vi "EstimateGamePiece2.vi"(7 "piece?":enum16{"None", "Cube", "Cone"}(ring), 9 "Confidence":dbl, 11 "Vision Timestamp (ms)":u32, 12 "Gamepiece Y":dbl, 13 "Gamepiece X":dbl, 14 "Vision Valid?":bool, 15 "Range":dbl) -> (8 "Seen_Game_Pieces":T1(array[cluster]))   [LabVIEW 2020]
uses:
  GlobalPoseAndTargeting.vi
  GlobalArm.vi
panel:
  in  "Acceptable Radius":dbl=5.0 format="%#_13g"
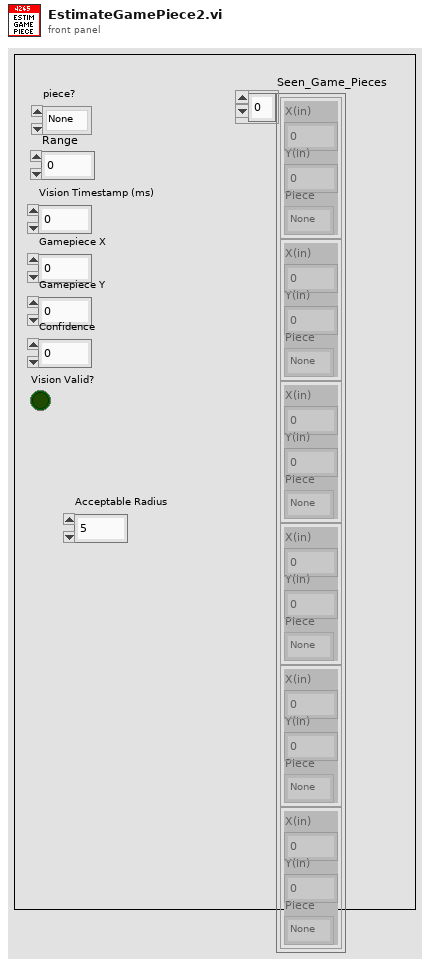
[diagram p1: front panel]
types:
  T1 = cluster{"X(in)":dbl, "Y(in)":dbl, "Piece":enum16{"None", "Cube", "Cone"}}[]
  T2 = cluster{"X":dbl, "Y":dbl, "Vision Timestamp (ms)":u32, "Confidence":dbl, "Range":dbl, "Piece":enum16{"None", "Cube", "Cone"}}
  T3 = cluster{"X":dbl, "Y":dbl, "Vision Timestamp (ms)":u32, "Confidence":dbl, "Range":dbl, "Piece":enum16{"None", "Cube", "Cone"}}[]
  T4 = cluster{"X(in)":dbl, "Y(in)":dbl, "Count":i32, "Timestamp(ms)":u32, "Piece":enum16{"None", "Cube", "Cone"}}
  T5 = cluster{"X(in)":dbl, "Y(in)":dbl, "Piece":enum16{"None", "Cube", "Cone"}}
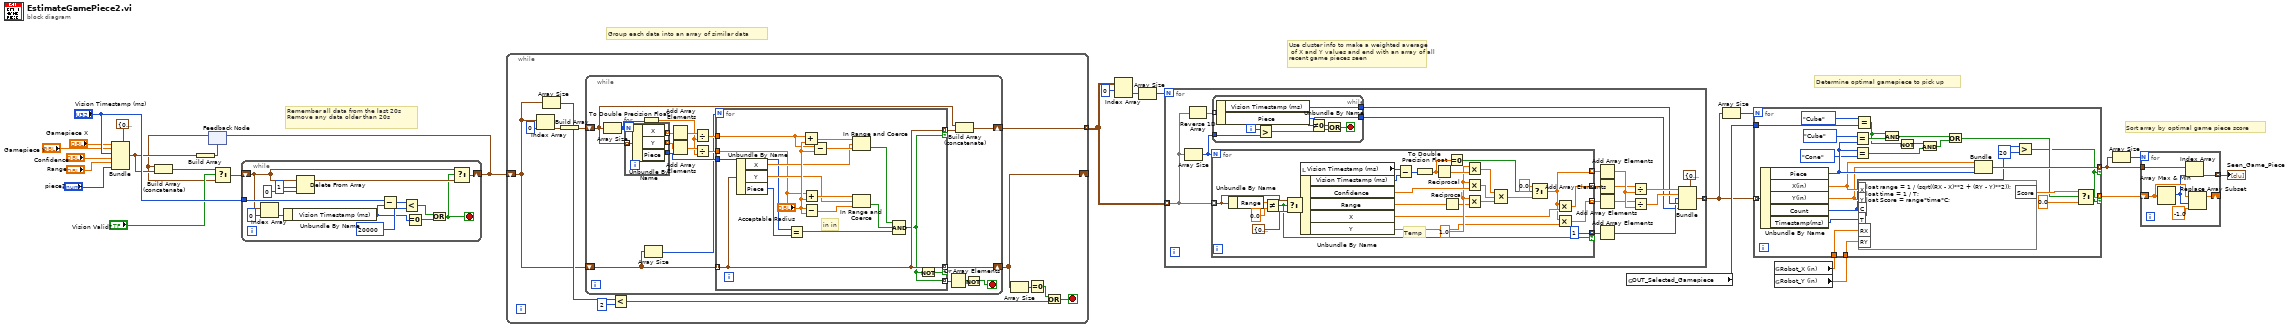
[diagram p0: block diagram]
diagram:
  # "Sort array by optimal game piece score"
  # "Determine optimal gamepiece to pick up"
  # "Use cluster info to make a weighted average\n of X and Y values and end with an array of all recent game pieces seen"
  # "Group each data into an array of similar data"
  # "Remember all data from the last 20s\nRemove any data older than 20s"
  n1 = Bundle(cluster=T2 {"X"=0.0, "Y"=0.0, "Vision Timestamp (ms)"=0, "Confidence"=0.0, "Range"=1.0, "Piece"=enum."None"} ("Cluster"), "X"="Gamepiece X", "Y"="Gamepiece Y", "Vision Timestamp (ms)"="Vision Timestamp (ms)", "Confidence"="Confidence", "Range"="Range", "Piece"="piece?") -> (w14:T2)
  n2 = Build Array(w14) -> (w13:T3)
  n3 = feedback #1(w13) -> (w2:T3)
  n4 = Build Array (concatenate)(w2, w14) -> (w4:T3)
  n5 = Select(t=w4, s="Vision Valid?", f=w2) -> (s? t:f=w5:T3)
  n6 = while {
    tunnel: "Vision Timestamp (ms)" -> [w39]
    shift-right: [w32] -> w1
    shift-left: w5 -> [w34]
    stop <- w28 stop-if-true
    n7 = Index Array(array=w34, index=0) -> (element=w40:T2)
    n8 = Unbundle By Name(w40) -> ("Vision Timestamp (ms)"=w31:u32)
    n9 = Delete From Array(array=w34, length=1, index=0) -> (array with subset deleted=w33:T3)  [unwired: 1 out]
    n10 = Subtract(x=w39, y=w31) -> (x-y=w38:u32)
    n11 = Less?(x=w38, y=u32 20000) -> (x < y?=w29:bool)
    n12 = Equal To 0?(x=w31) -> (x = 0?=w30:bool)
    n13 = Or(x=w29, y=w30) -> (x .or. y?=w28:bool)
    n14 = Select(t=w34, s=w28, f=w33) -> (s? t:f=w32:T3)
  }
  n15 = feedback-in #1(w1) -> ()
  n16 = while {
    shift-right: [w42] -> _
    shift-left: w1 -> [w46]
    tunnel: [w43] -> w11 mode=indexing
    stop <- w49 stop-if-true
    n17 = Index Array(array=w46, index=0) -> (element=w45:T2)
    n18 = Array Size(array=w46) -> (size(s)=w52:i32)
    n19 = Build Array(w45) -> (w44:T3)
    n20 = while {
      shift-right: [w62] -> w42
      shift-left: w46 -> [w55]
      shift-right: [w59] -> w43
      shift-left: w44 -> [w60]
      stop <- w56 stop-if-true
      n21 = Array Size(array=w60) -> (size(s)=w66:i32)
      n22 = for {
        N: w66 -> [_]
        tunnel: w60 -> [w75] mode=indexing
        tunnel: [w74] -> w71 mode=indexing
        tunnel: [w73] -> w70 mode=indexing
        tunnel: [w72] -> w69
        n23 = Unbundle By Name(w75) -> ("X"=w74:dbl, "Y"=w73:dbl, "Piece"=w72:enum16{"None", "Cube", "Cone"})
      }
      n24 = To Double Precision Float(number=w66) -> (double precision float=w63:dbl)
      n25 = Array Size(array=w55) -> (size(s)=w54:i32)
      n26 = Add Array Elements(numeric array=w71) -> (sum=w67:dbl)
      n27 = Add Array Elements(numeric array=w70) -> (sum=w65:dbl)
      n28 = Divide(x=w67, y=w63) -> (x/y=w68:dbl)
      n29 = Divide(x=w65, y=w63) -> (x/y=w64:dbl)
      n30 = for {
        N: w54 -> [_]
        tunnel: w55 -> [w80] mode=indexing
        tunnel: [w80] -> w61 mode=indexing if=w76
        tunnel: [w80] -> w62 mode=indexing if=w81
        tunnel: w68 -> [w79]
        tunnel: w64 -> [w78]
        tunnel: w69 -> [w77]
        tunnel: [w76] -> w58 mode=indexing
        # "in in"
        n31 = Unbundle By Name(w80) -> ("X"=w82:dbl, "Y"=w83:dbl, "Piece"=w84:enum16{"None", "Cube", "Cone"})
        n32 = Equal?(x=w77, y=w84) -> (x = y?=w85:bool)
        n33 = Add(x=w79, y="Acceptable Radius") -> (x+y=w92:dbl)
        n34 = Add(x=w78, y="Acceptable Radius") -> (x+y=w90:dbl)
        n35 = Subtract(x=w78, y="Acceptable Radius") -> (x-y=w89:dbl)
        n36 = Subtract(x=w79, y="Acceptable Radius") -> (x-y=w91:dbl)
        n37 = In Range and Coerce(upper limit=w92, x=w82, lower limit=w91) -> (In Range?=w87:bool)  [unwired: 1 out]
        n38 = In Range and Coerce(upper limit=w90, x=w83, lower limit=w89) -> (In Range?=w86:bool)  [unwired: 1 out]
        n39 = Compound Arithmetic op=AND(w87, w86, w85) -> (w76:bool)
        n40 = Not(x=w76) -> (.not. x?=w81:bool)
      }
      n41 = Or Array Elements(Boolean array=w58) -> (logical OR=w57:bool)
      n42 = Build Array (concatenate)(w60, w61) -> (w59:T3)
      n43 = Not(x=w57) -> (.not. x?=w56:bool)
    }
    n44 = Less?(x=w52, y=2) -> (x < y?=w48:bool)
    n45 = Array Size(array=w42) -> (size(s)=w53:i32)
    n46 = Equal To 0?(x=w53) -> (x = 0?=w50:bool)
    n47 = Or(x=w50, y=w48) -> (x .or. y?=w49:bool)
  }
  n48 = Index Array(array=w11, index (row)=0) -> (element=w25:T3)  [unwired: 1 in]
  n49 = Array Size(array=w25) -> (size(s)=w26:i32)
  n50 = for {
    N: w26 -> [_]
    tunnel: w11 -> [w94] mode=indexing
    tunnel: [w105] -> w19 mode=indexing
    n51 = Array Size(array=w94) -> (size(s)=w93:i32)
    n52 = Reverse 1D Array(array=w94) -> (reversed array=w98:T3)
    n53 = for {
      N: w93 -> [_]
      tunnel: w94 -> [w124] mode=indexing
      tunnel: [w119] -> w104 mode=indexing
      tunnel: [w131] -> w102 mode=indexing
      tunnel: [w120] -> w100 mode=indexing
      tunnel: [1] -> w97 mode=indexing if=w118
      w139 = 1.0 ("x")
      # "Temp"
      n54 = Unbundle By Name(w124) -> ("Range"=w127:dbl)
      n55 = Not Equal?(x=w127, y=0.0) -> (x != y?=w118:bool)
      n56 = Select(t=w124, s=w118, f=T2 {"X"=0.0, "Y"=0.0, "Vision Timestamp (ms)"=1, "Confidence"=0.0, "Range"=1.0, "Piece"=enum."None"} ("Cluster")) -> (s? t:f=w123:T2)
      n57 = local read "Vision Timestamp (ms)"() -> (w143:u32)
      n58 = Unbundle By Name(w123) -> ("Vision Timestamp (ms)"=w144:u32, "Confidence"=w141:dbl, "Range"=w130:dbl, "X"=w137:dbl, "Y"=w136:dbl)
      n59 = Subtract(x=w143, y=w144) -> (x-y=w135:u32)
      n60 = To Double Precision Float(number=w135) -> (double precision float=w122:dbl)
      n61 = Reciprocal(x=w122) -> (1/x=w142:dbl)
      n62 = Reciprocal(x=w130) -> (1/x=w134:dbl)
      n63 = Equal To 0?(x=w122) -> (x = 0?=w133:bool)
      n64 = Multiply(x=w139, y=w142) -> (x*y=w129:dbl)
      n65 = Multiply(x=w139, y=w141) -> (x*y=w140:dbl)
      n66 = Multiply(x=w139, y=w134) -> (x*y=w138:dbl)
      n67 = Compound Arithmetic op=MULTIPLY(w129, w140, w138) -> (w128:dbl)
      n68 = Select(t=0.0, s=w133, f=w128) -> (s? t:f=w119:dbl)
      n69 = Multiply(x=w119, y=w137) -> (x*y=w120:dbl)
      n70 = Multiply(x=w119, y=w136) -> (x*y=w131:dbl)
    }
    n71 = while {
      tunnel: [w116] -> w107
      tunnel: w98 -> [w117] mode=indexing
      tunnel: [w115] -> w95
      tunnel: w93 -> [w113]
      i -> [w114]
      stop <- w112 stop-if-true
      n72 = Unbundle By Name(w117) -> ("Vision Timestamp (ms)"=w116:u32, "Piece"=w115:enum16{"None", "Cube", "Cone"})
      n73 = Greater?(x=w114, y=w113) -> (0:w110:bool)
      n74 = Not Equal To 0?(x=w116) -> (x != 0?=w111:bool)
      n75 = Or(x=w111, y=w110) -> (x .or. y?=w112:bool)
    }
    n76 = Add Array Elements(numeric array=w104) -> (sum=w103:dbl)
    n77 = Add Array Elements(numeric array=w100) -> (sum=w99:dbl)
    n78 = Add Array Elements(numeric array=w102) -> (sum=w101:dbl)
    n79 = Add Array Elements(numeric array=w97) -> (sum=w96:i32)
    n80 = Divide(x=w99, y=w103) -> (x/y=w109:dbl)
    n81 = Divide(x=w101, y=w103) -> (x/y=w108:dbl)
    n82 = Bundle(cluster=T4 {"X(in)"=0.0, "Y(in)"=0.0, "Count"=0, "Timestamp(ms)"=0, "Piece"=enum."None"}, "X(in)"=w109, "Y(in)"=w108, "Count"=w96, "Timestamp(ms)"=w107, "Piece"=w95) -> (w105:T4)
  }
  n83 = global read "GlobalArm.vi" "OUT_Selected_Gamepiece"() -> (w20:enum16{"Cube", "Cone"})
  n84 = Array Size(array=w19) -> (size(s)=w24:i32)
  n85 = global read "GlobalPoseAndTargeting.vi" "Robot_X (in)"() -> (w22:dbl)
  n86 = global read "GlobalPoseAndTargeting.vi" "Robot_Y (in)"() -> (w21:dbl)
  n87 = for {
    N: w24 -> [_]
    tunnel: w19 -> [w169] mode=indexing
    tunnel: w22 -> [w153]
    tunnel: w21 -> [w152]
    tunnel: w20 -> [w167]
    tunnel: [w149] -> w17 mode=indexing if=w145
    tunnel: [w168] -> w16 mode=indexing if=w145
    n88 = Unbundle By Name(w169) -> ("Piece"=w161:enum16{"None", "Cube", "Cone"}, "X(in)"=w156:dbl, "Y(in)"=w155:dbl, "Count"=w148:i32, "Timestamp(ms)"=w154:u32)
    n89 = Equal?(x=enum16{"None", "Cube", "Cone"}."Cube", y=w161) -> (x = y?=w162:bool)
    n90 = Equal?(x=w161, y=enum16{"None", "Cube", "Cone"}."Cone" ("x")) -> (x = y?=w159:bool)
    n91 = Equal?(x=enum16{"Cube", "Cone"}."Cube", y=w167) -> (x = y?=w157:bool)
    n92 = formula code="float range = 1 / (sqrt((RX - X)**2 + (RY - Y)**2));\nfloat time = 1 / T;\nfloat Score = range*time*C;"("X"=w156, "Y"=w155, "C"=w148, "T"=w154, "RY"=w152, "RX"=w153) -> ("Score"=w150:dbl)
    n93 = And(x=w157, y=w162) -> (x .and. y?=w164:bool)
    n94 = Not(x=w157) -> (.not. x?=w158:bool)
    n95 = And(x=w158, y=w159) -> (x .and. y?=w163:bool)
    n96 = Or(x=w164, y=w163) -> (x .or. y?=w146:bool)
    n97 = Bundle("X(in)"=w156, "Y(in)"=w155, "Piece"=w161) -> (w168:T5)  [unwired: 1 in]
    n98 = Greater?(x=w148, y=20) -> (0:w145:bool)
    n99 = Select(t=w150, s=w146, f=0.0) -> (s? t:f=w149:dbl)
  }
  n100 = Array Size(array=w16) -> (size(s)=w18:i32)
  n101 = for {
    N: w18 -> [_]
    tunnel: w16 -> [w175]
    shift-right: [w173] -> _
    shift-left: w17 -> [w172]
    tunnel: [w174] -> w12 mode=indexing
    n102 = Array Max & Min(array=w172) -> (max index (indices)=w170:i32)  [unwired: 3 out]
    n103 = Index Array(array=w175, index=w170) -> (element=w174:T5)
    n104 = Replace Array Subset(array=w172, new element=-1.0 ("new element/subarray"), index=w170) -> (w173:dbl[])
  }
  "Seen_Game_Pieces" <- w12
